vi "test.vi"   [LabVIEW 2014]
uses:
  LabView/Create Dataset 2D Integer.vi
  LabView/Append To Dataset 2D Integer.vi
  LabView/HDF5Tools.lvlib
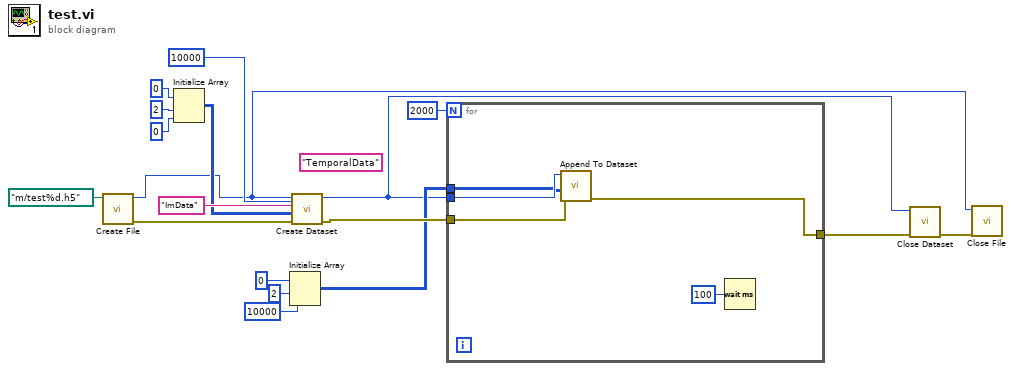
[diagram p0: block diagram]
diagram:
  (unwired) "TemporalData" ("Dataset name")
  n1 = call "Create File.vi"("File Name"=path "m:/test%d.h5") -> ("Error out"=w15:errorcluster, "file_id"=w1:i32)  [unwired: 7 in]
  n2 = Initialize Array(0, 2 ("dimension size"), 0 ("dimension size")) -> (w13:i32[][])
  n3 = Initialize Array(0 ("element"), 2 ("dimension size"), 10000 ("dimension size")) -> (w5:i32[][])
  n4 = call-poly "Create Dataset.vi"("Chunk size"=10000, "error in (no error)"=w15, "Datatype"=w13, "Dataset name"="ImData", "Location id in"=w1) -> ("error out"=w10:errorcluster, "Dataset id"=w3:i32)  [unwired: 5 in]
  n5 = for {
    N: 2000 -> [_]
    tunnel: w3 -> [w23]
    tunnel: w10 -> [w22]
    tunnel: w5 -> [w21]
    tunnel: [w20] -> w4
    n6 = call-poly "Append To Dataset.vi"("error in (no error)"=w22, "data"=w21, "dataset_id"=w23) -> ("error out"=w20:errorcluster)  [unwired: 7 in, 1 out]
    n7 = Wait (ms)(milliseconds to wait=u32 100) -> ()  [unwired: 1 out]
  }
  n8 = call "Close Dataset.vi"("error in (no error)"=w4, "dataset_id"=w3) -> ("error out"=w2:errorcluster)  [unwired: 9 in]
  n9 = call "Close File.vi"("error in (no error)"=w2, "file_id"=w1) -> ()  [unwired: 9 in, 1 out]
